vi "Write Stack Plots.vi"(8 "error in (no error)":errorcluster, 10 "StackPlots":bool, 11 "WaveformChart.lvclass in":refnum<class "WaveformChart.lvclass">) -> (0 "error out":errorcluster, 3 "WaveformChart.lvclass out":refnum<class "WaveformChart.lvclass">)   [LabVIEW 2015, in "WaveformChart.lvclass"]
uses:
  WaveformChart.lvclass
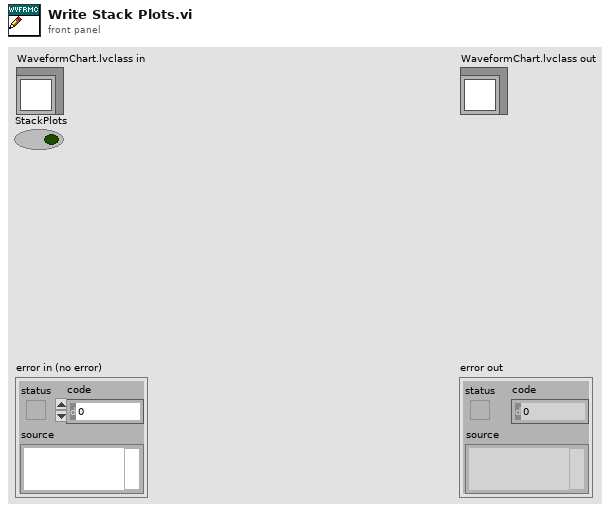
[diagram p1: front panel]
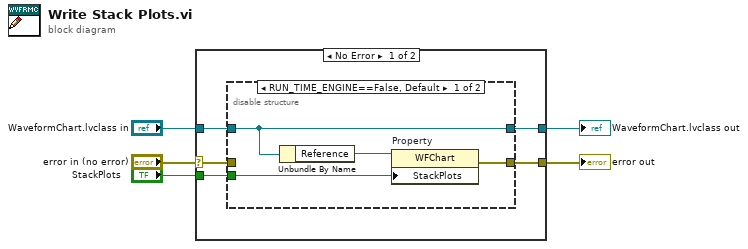
[diagram p0: block diagram]
diagram:
  n1 = case shown="No Error" "error in (no error)" {
    selector: "error in (no error)" -> [w6 w18]
    tunnel: [w10 w18] -> w4
    tunnel: [w7 w17] -> w2
    tunnel: "WaveformChart.lvclass in" -> [w8 w17]
    tunnel: "StackPlots" -> [w9 _]
    frame No Error {
      n2 = disable-structure shown="RUN_TIME_ENGINE==False, Default" {
        disable-tunnel: [w14 w15] -> w10
        disable-tunnel: w9 -> [w13 _]
        disable-tunnel: w8 -> [w11 w16]
        disable-tunnel: [w11 w16] -> w7
        disable-tunnel: w6 -> [_ w15]
        frame condition #0 (active) {
          n3 = Unbundle By Name(w11) -> ("Reference"=w12:refnum<vi>)
          n4 = property on="Property" class="WFChart"(reference=w12, "StackPlots"=w13) -> (error out=w14:errorcluster)  [unwired: 1 in, 1 out]
        }
        frame condition #1 {
        }
      }
    }
    frame Error {
    }
  }
  "error out" <- w4
  "WaveformChart.lvclass out" <- w2
